vi "Page Log.vi"(10 "Variables in":map{string, string[]}(c390), 11 "Request":T1) -> (0 "Content-Type":string, 1 "Content":string, 2 "Headers":map{string, string}(c390), 3 "Status":i32)   [LabVIEW 2021, in "HttpServer.lvlib"]
uses:
  HttpServer.lvlib
  TypeDefs/Request.ctl
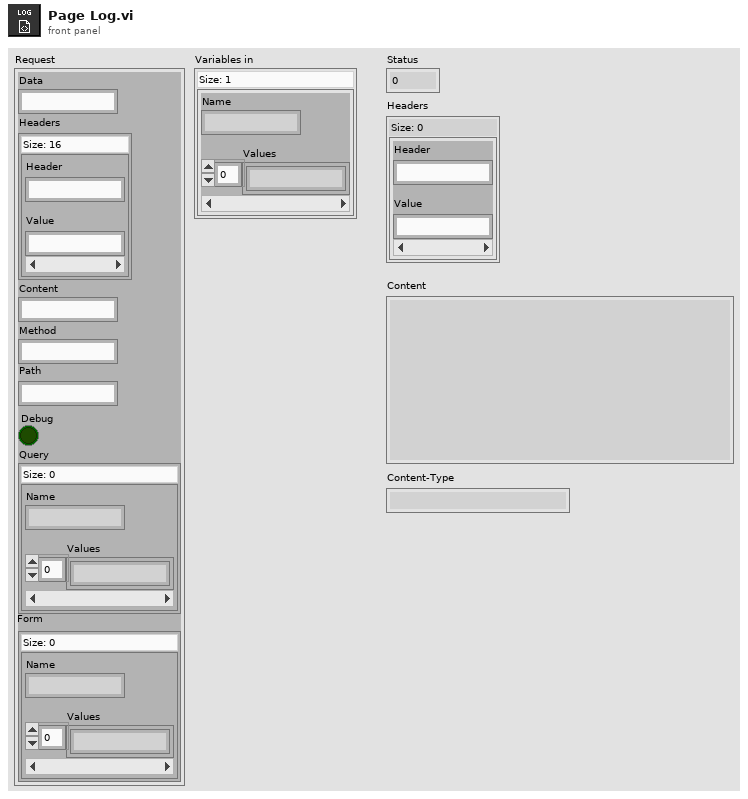
[diagram p1: front panel]
types:
  T1 = typedef "HttpServer.lvlib/Request.ctl" = cluster{"Data":string, "Headers":map{string, string}, "Content":string, "Method":string, "Path":string, "Debug":bool, "Query":map{string, string[]}, "Form":map{string, string[]}}
  T2 = cluster{"time":timestamp, "error":errorcluster}[]
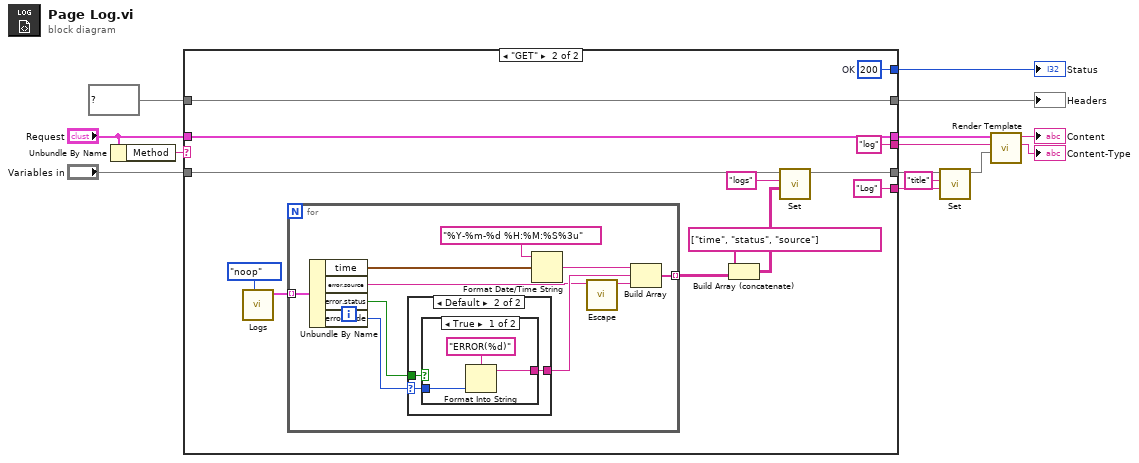
[diagram p0: block diagram]
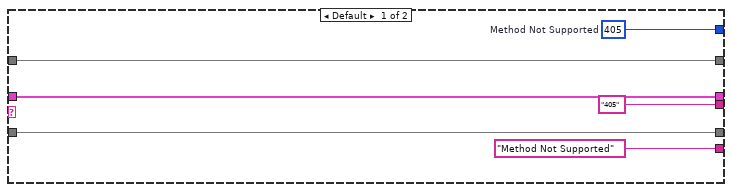
[diagram p2: hidden frame]
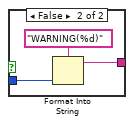
[diagram p4: hidden frame]
diagram:
  n1 = Unbundle By Name("Request") -> ("Method"=w12:string)
  n2 = case shown="\"GET\"" w12 {
    tunnel: "Variables in" -> [w18 w28]
    tunnel: [w20 w33] -> w4
    tunnel: [w19 w32] -> w8
    tunnel: "Request" -> [w19 w32]
    tunnel: ["Method Not Supported" "Log"] -> w11
    tunnel: [w18 w26] -> w10
    tunnel: ["405" "log"] -> w7
    tunnel: [w17 w24] -> w2
    tunnel: map{string, string} {} ("Headers") -> [w17 w24]
    frame Default {
      w20 = 405  # Method Not Supported
    }
    frame "GET" {
      w33 = 200  # OK
      n3 = call "Logs.vi"("Action"=enum8{"noop", "add", "clear"}."noop") -> ("logs"=w29:T2)  [unwired: 10 in]
      n4 = for {
        tunnel: w29 -> [w43] mode=indexing
        tunnel: [w36] -> w23 mode=indexing
        n5 = Unbundle By Name(w43) -> ("time"=w42:timestamp, "error.source"=w35:string, "error.status"=w40:bool, "error.code"=w39:i32)
        n6 = case shown="Default" w39 {
          selector: w39 -> [_ w45]
          tunnel: w40 -> [_ w46]
          tunnel: [_ w44] -> w37
          frame 0 {
          }
          frame Default {
            n7 = case shown="True" w46 {
              tunnel: w45 -> [w49 w52]
              tunnel: [w47 w50] -> w44
              frame True {
                n8 = Format Into String(format string="ERROR(%d)", w49) -> (resulting string=w47:string)  [unwired: 2 in, 1 out]
              }
              frame False {
                n9 = Format Into String(format string="WARNING(%d)", w52) -> (resulting string=w50:string)  [unwired: 2 in, 1 out]
              }
            }
          }
        }
        n10 = Format Date/Time String(time format string (%c)="%Y-%m-%d %H:%M:%S%3u", seconds (now)=w42) -> (date/time string=w38:string)  [unwired: 1 in]
        n11 = call "Escape.vi"("text"=w35) -> ("escaped text"=w34:string)  [unwired: 10 in]
        n12 = Build Array(w38, w37, w34) -> (w36:string[])
      }
      n13 = Build Array (concatenate)(string[] ["time", "status", "source"], w23) -> (w22:string[][])
      n14 = call "Set.vi"("Value [Scalar, Cluster, 1D_Clusters, 2D_String]"=w22, "Name"="logs" ("Variable[.Key]"), "Variables in"=w28) -> ("Variables out"=w26:map{string, string[]})  [unwired: 7 in, 1 out]
    }
  }
  "Status" <- w4
  "Headers" <- w2
  n15 = call "Set.vi"("Value [Scalar, Cluster, 1D_Clusters, 2D_String]"=w11, "Name"="title" ("key"), "Variables in"=w10) -> ("Variables out"=w6:map{string, string[]})  [unwired: 7 in, 1 out]
  n16 = call "Render Template.vi"("Variables in"=w6, "Endpoint"=w7, "Request"=w8) -> ("Content-Type"=→"Content-Type":string, "Content out"=→"Content":string)  [unwired: 7 in]
